vi "Toggle With Reset.vi"(6 "Reset":bool, 10 "Toggle":bool) -> (2 "Output":bool)   [LabVIEW 2016]
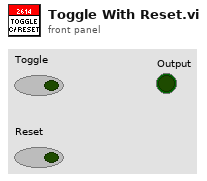
[diagram p1: front panel]
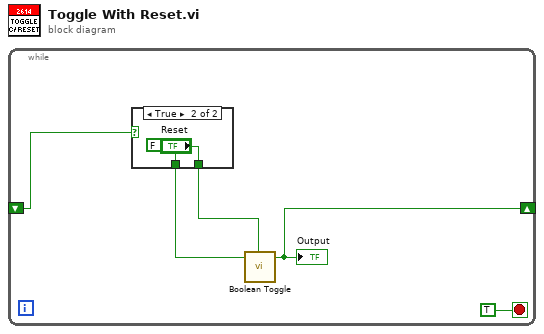
[diagram p0: block diagram]
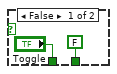
[diagram p2: hidden frame]
diagram:
  n1 = while {
    shift-right: [w4] -> _
    shift-left: _ -> [w3]
    stop <- TRUE stop-if-true
    n2 = case shown="True" w3 {
      tunnel: [FALSE ("Reset") "Reset"] -> w2
      tunnel: ["Toggle" FALSE ("Toggle")] -> w1
      frame False {
      }
      frame True {
      }
    }
    n3 = call "Boolean Toggle.vi"("Input"=w1, "Reset"=w2) -> ("Output"=w4:bool)  [unwired: 25 in]
    "Output" <- w4
  }
